vi "Fire Private Event.vi"(7 "AdHoc Cmd (\"\")":string, 8 "error in (no error)":errorcluster, 9 "vData":variant, 10 "PrivAsyncCmd":T1, 11 "DAQ_Engine in":refnum<class "DAQ_Engine.lvclass">) -> (0 "error out":errorcluster, 3 "DAQ_Engine out":refnum<class "DAQ_Engine.lvclass">)   [LabVIEW 2019, in "DAQ_Engine.lvclass"]
doc: "Developed by Kevin Thompson\nkevin@thompsonengineering.net\n\nCopyright 2018\nThompson Engineering, LLC"
uses:
  DAQ_Engine.lvclass
  Common/DataTypes/TD Async CmdMsg EventData--cluster.ctl
  DataTypes/PrivateAsynEv_DAQ_Engine--enum.ctl
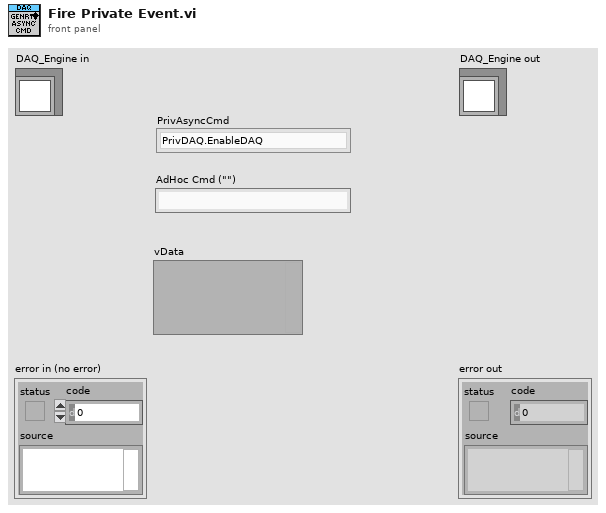
[diagram p1: front panel]
types:
  T1 = typedef "DAQ_Engine.lvclass/PrivateAsynEv_DAQ_Engine--enum.ctl" = enum16{"PrivDAQ.EnableDAQ", "PrivDAQ.ClearDAQError"}
  T2 = typedef "TD Async CmdMsg EventData--cluster.ctl" = cluster{"Time Stamp":timestamp, "CmdMsg":string, "vData":variant}
  T3 = typedef "DAQ_Engine.lvclass/ObjData--cluster.ctl" = cluster{"Settings":T4, "Public Events":T9, "Dependency":T10, "ReadData-placeholder":T11, "VISA-placeholder":refnum<visa-resource-name>, "MeasSettings":T5, "InverterDataAcqMode":T8, "RawDaqDataQ":T12, "Private Events":T13, "DAQState Data":T14}
  T4 = typedef "DAQ_Engine.lvclass/Settings--cluster.ctl" = cluster{"Simulation":bool, "Initial ErrReporting setting":i32, "Initial Measurement settings":T5, "BoardNum":T7, "Acquisition mode":T8, "DemoMode":bool}
  T5 = typedef "Measurement Config--cluster.ctl" = cluster{"Data Rate 9775":T6, "Data Rate 9215":u32, "Samples RMS 9215":u32, "Samples RMS 9775":u32}
  T6 = typedef "nicrio_cRIO-9775_ContinuousDataRates4ChansRing.ctl" = u16
  T7 = typedef "DAQ_Engine.lvclass/BoardNum--cluster.ctl" = cluster{"P1Sgl":u32, "P2":u32, "P3":u32}
  T8 = typedef "Acquisition Mode--cluster.ctl" = enum16{"3phase", "Single"}
  T9 = typedef "DAQ_Engine.lvclass/Public Events--cluster.ctl" = cluster{"DAQ_Engine.AsyncCmd Event":refnum<user-event>, "DAQ_Engine.AsyncMsg Event":refnum<user-event>, "stop process":refnum<user-event>, "DAQ_Engine.DAQStateChg Ev":refnum<user-event>, "DAQ_Engine.MeasSettingsChg Ev":refnum<user-event>, "DAQ_Engine.AcqModeChg Ev":refnum<user-event>}
  T10 = typedef "DAQ_Engine.lvclass/Dependency--cluster.ctl" = cluster{"Config":refnum<class "Config.lvclass">}
  T11 = typedef "DAQ_Engine.lvclass/Read Data--cluster.ctl" = cluster{"Data":dbl}
  T12 = typedef "RawDAQDataQRef--cluster.ctl" = refnum<queue>
  T13 = typedef "DAQ_Engine.lvclass/Private Events--cluster.ctl" = cluster{"PrivateAsync Ev":refnum<user-event>}
  T14 = typedef "DAQ_Engine.lvclass/DAQStateEvData--cluster.ctl" = cluster{"DAQState":T15, "vData":variant}
  T15 = typedef "DAQState--enum.ctl" = enum16{"Unknown", "Stopped", "Running", "Error"}
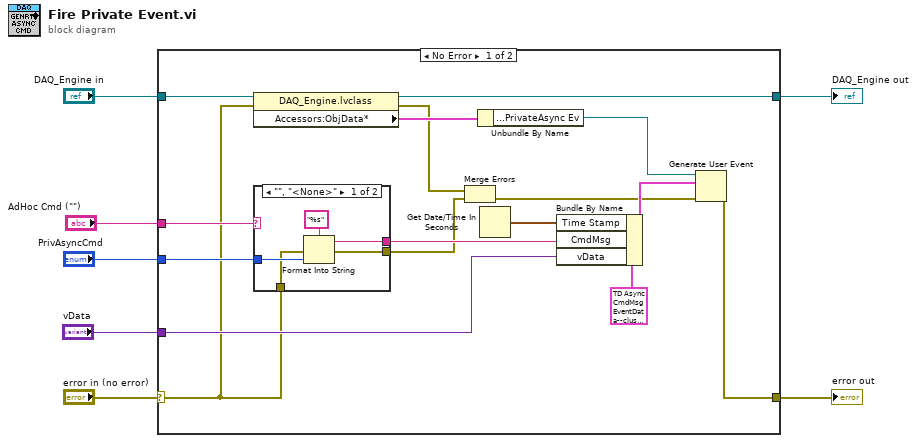
[diagram p0: block diagram]
diagram:
  n1 = case shown="No Error" "error in (no error)" {
    selector: "error in (no error)" -> [w9 w32]
    tunnel: [w23 w32] -> w6
    tunnel: [w13 w31] -> w4
    tunnel: "DAQ_Engine in" -> [w14 w31]
    tunnel: "PrivAsyncCmd" -> [w17 _]
    tunnel: "vData" -> [w18 _]
    tunnel: "AdHoc Cmd (\"\")" -> [w16 _]
    frame No Error {
      n2 = property class="DAQ_Engine.lvclass"(reference=w14, error in=w9) -> (reference out=w13:refnum<class "DAQ_Engine.lvclass">, error out=w10:errorcluster, "Accessors:ObjData*"=w15:T3)
      n3 = case shown="\"\", \"<None>\"" w16 {
        selector: w16 -> [_ w29]
        tunnel: w17 -> [w27 _]
        tunnel: [w26 w29] -> w19
        tunnel: w9 -> [w25 w30]
        tunnel: [w24 w30] -> w12
        frame "", "<None>" {
          n4 = Format Into String(format string="%s", error in=w25, w27) -> (resulting string=w26:string, error out=w24:errorcluster)  [unwired: 1 in]
        }
        frame Default {
        }
      }
      n5 = Merge Errors(w10, w12) -> (w11:errorcluster)
      n6 = Unbundle By Name(w15) -> ("Private Events.PrivateAsync Ev"=w8:refnum<user-event>)
      n7 = Get Date/Time In Seconds() -> (seconds since 1Jan1904=w20:timestamp)
      n8 = Bundle By Name(cluster=T2 {"Time Stamp"=timestamp(0 s since 1904-01-01), "CmdMsg"="", "vData"=variant} ("Async EvData"), "Time Stamp"=w20, "CmdMsg"=w19, "vData"=w18) -> (w22:T2)
      n9 = Generate User Event(user event=w8, event data cluster=w22, error in=w11) -> (error out=w23:errorcluster)  [unwired: 1 in, 1 out]
    }
    frame Error {
    }
  }
  "error out" <- w6
  "DAQ_Engine out" <- w4
